vi "controlAQuadBInResolution.vi"(6 "Set":bool, 7 "error in":errorcluster, 8 "Resolution in":i32, 9 "axis in":u8, 10 "connection ID":refnum<k5>) -> (0 "error out":errorcluster, 1 "Resolution out":i32, 2 "axis out":u8, 3 "connection ID":refnum<k5>)   [LabVIEW 2016]
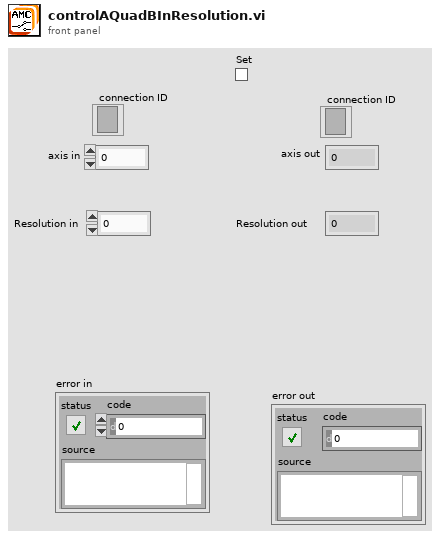
[diagram p1: front panel]
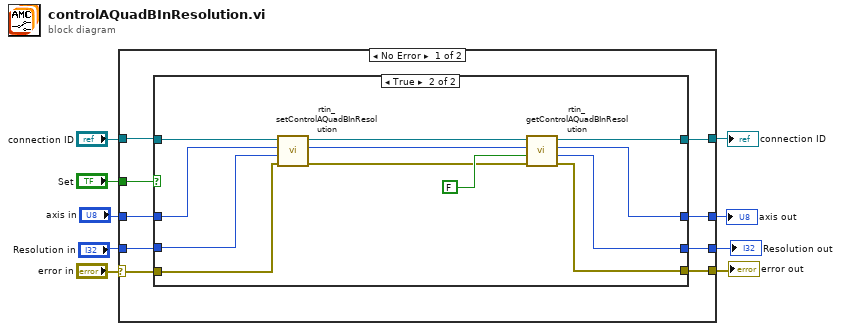
[diagram p0: block diagram]
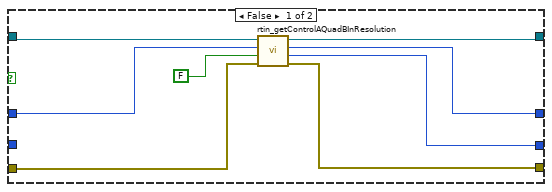
[diagram p2: hidden frame]
diagram:
  n1 = case shown="No Error" "error in" {
    selector: "error in" -> [w12 w42]
    tunnel: "axis in" -> [w16 w40]
    tunnel: [w14 w42] -> w8
    tunnel: [w11 w40] -> w7
    tunnel: "Set" -> [w13 _]
    tunnel: [w17 w39] -> w5
    tunnel: "connection ID" -> [w18 w39]
    tunnel: "Resolution in" -> [w15 w41]
    tunnel: [w10 w41] -> w3
    frame No Error {
      n2 = case shown="True" w13 {
        tunnel: [w25 w32] -> w17
        tunnel: w18 -> [w26 w38]
        tunnel: w16 -> [w22 w37]
        tunnel: [w23 w29] -> w14
        tunnel: w15 -> [_ w36]
        tunnel: w12 -> [w24 w35]
        tunnel: [w21 w27] -> w11
        tunnel: [w20 w28] -> w10
        frame False {
          n3 = call "rtin_getControlAQuadBInResolution.vi"("error in"=w24, "tempvalue"=FALSE, "axis"=w22, "connection ID"=w26) -> ("error out"=w23:errorcluster, "resolution"=w20:i32, "axis_out"=w21:i32, "connection ID"=w25:refnum<k5>)  [unwired: 4 in]
        }
        frame True {
          n4 = call "rtin_setControlAQuadBInResolution.vi"("error in"=w35, "resolution"=w36, "axis"=w37, "connection ID"=w38) -> ("error out"=w30:errorcluster, "axis_out"=w31:i32, "connection ID"=w33:refnum<k5>)  [unwired: 5 in]
          n5 = call "rtin_getControlAQuadBInResolution.vi"("error in"=w30, "tempvalue"=FALSE, "axis"=w31, "connection ID"=w33) -> ("error out"=w29:errorcluster, "resolution"=w28:i32, "axis_out"=w27:i32, "connection ID"=w32:refnum<k5>)  [unwired: 4 in]
        }
      }
    }
    frame Error {
    }
  }
  "error out" <- w8
  "axis out" <- w7
  "connection ID" <- w5
  "Resolution out" <- w3
